vi "SMC_GetPos.vi"(8 "error in (no error)":errorcluster) -> (0 "error out":errorcluster, 3 "Answer":string)   [LabVIEW 2015]
uses:
  SMC_SubVIs.llb/SMC_ManagerMode.ctl
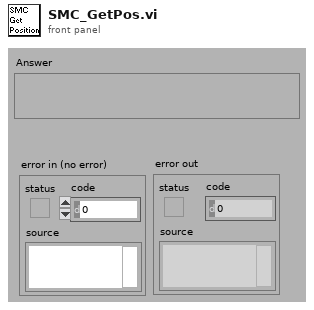
[diagram p1: front panel]
types:
  T1 = typedef "SMC_ManagerMode.ctl" = enum16{"Init", "Get", "SetPosition", "SetStatus", "SetMoving", "SetControllerNr"}
  T2 = typedef "SMC Paras.ctl" = cluster{"VENUS Language":T3, "Number of Axis":u8, "Controller Nr":u8, "Simulation":bool}
  T3 = typedef "VENUSNr.ctl" = enum16{"VENUS 2", "VENUS 1"}
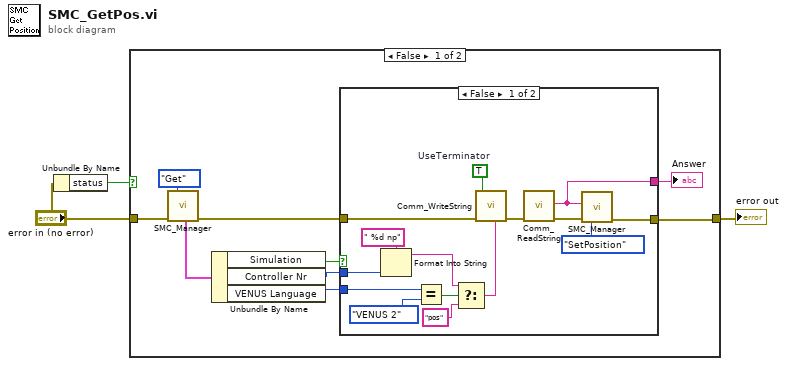
[diagram p0: block diagram]
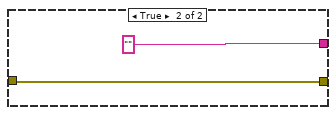
[diagram p2: hidden frame]
diagram:
  n1 = Unbundle By Name("error in (no error)") -> ("status"=w3:bool)
  n2 = case shown="False" w3 {
    tunnel: "error in (no error)" -> [w9 w30]
    tunnel: [w10 w30] -> w1
    frame False {
      n3 = call "SMC_Manager.vi"("Mode"=SMC_ManagerMode."Get", "error in (no error)"=w9) -> ("SMC Parameter Out"=w6:T2, "error out"=w8:errorcluster)  [unwired: 9 in, 3 out]
      n4 = Unbundle By Name(w6) -> ("Simulation"=w4:bool, "Controller Nr"=w5:u8, "VENUS Language"=w7:T3)
      n5 = case shown="False" w4 {
        tunnel: [w26 "" ("Answer")] -> w11
        tunnel: [w25 w29] -> w10
        tunnel: w8 -> [w24 w29]
        tunnel: w7 -> [w20 _]
        tunnel: w5 -> [w18 _]
        frame False {
          w13 = TRUE  # UseTerminator
          n6 = Format Into String(format string=" %d np" ("Format String"), w18) -> (resulting string=w17:string)  [unwired: 2 in, 1 out]
          n7 = Equal?(x=w20, y=enum16{"VENUS 2", "VENUS 1"}."VENUS 2") -> (x = y?=w15:bool)
          n8 = Select(t=w17, s=w15, f="pos" ("string to write")) -> (s? t:f=w14:string)
          n9 = call "Comm_WriteString.vi"("string to write"=w14, "error in (no error)"=w24, "UseTerminator"=w13) -> ("error out"=w21:errorcluster)  [unwired: 8 in]
          n10 = call "Comm_ReadString.vi"("error in (no error)"=w21) -> ("error out"=w23:errorcluster, "Answer"=w26:string)  [unwired: 9 in]
          n11 = call "SMC_Manager.vi"("Mode"=SMC_ManagerMode."SetPosition", "error in (no error)"=w23, "String In"=w26) -> ("error out"=w25:errorcluster)  [unwired: 8 in, 4 out]
        }
        frame True {
        }
      }
      "Answer" <- w11
    }
    frame True {
      # "Error, do nothing"
    }
  }
  "error out" <- w1
